vi "UIManager.Init.vi"(6 "JQMHStartup in":refnum<class "ModuleStartup.lvclass">, 8 "error in (no error)":errorcluster, 11 "NewTemplate in":refnum<class "UIManager.lvclass">) -> (0 "error out":errorcluster, 1 "StartupParams":variant, 2 "Requests":T2, 3 "NewTemplate out":refnum<class "UIManager.lvclass">, 4 "JQMHStartup out":refnum<class "ModuleStartup.lvclass">, 5 "StandardRequests":refnum<event-registration>)   [LabVIEW 2024, in "UIManager.lvclass"]
uses:
  UIManager.lvclass
  UIManager.lvclass/UIManager.ctl
  C:/Git/JA/JQMH/RQMHCore/ModuleCore/Module.lvclass
  C:/Git/JA/JQMH/ModuleTemplates/UIManager/UIManager.lvclass
  RQMHCore/Shared/ModuleShared.lvlib
  RQMHCore/ModuleCore/Module.lvclass
  RQMHCore/Startup/ModuleStartup.lvclass
  RQMHCore/ModuleCore/StopEventArgs.ctl
  Request Events--cluster.ctl
  RQMHCore/ModuleCore/StandardRequests.ctl
  RQMHCore/ModuleCore/Show Front Panel--Args.ctl
  RQMHCore/ModuleCore/Hide Front Panel.ctl
  RQMHCore/ModuleCore/Show Block Diagram.ctl
  RQMHCore/ModuleCore/Hide Block Diagram--Args.ctl
  RQMHCore/ModuleCore/Reply.ctl
  Do Something Args.ctl
  RQMHCore/ModuleCore/InitialiseArgs.ctl
  Prepare Args.ctl
  Show Args.ctl
  Add Eng Panel Args.ctl
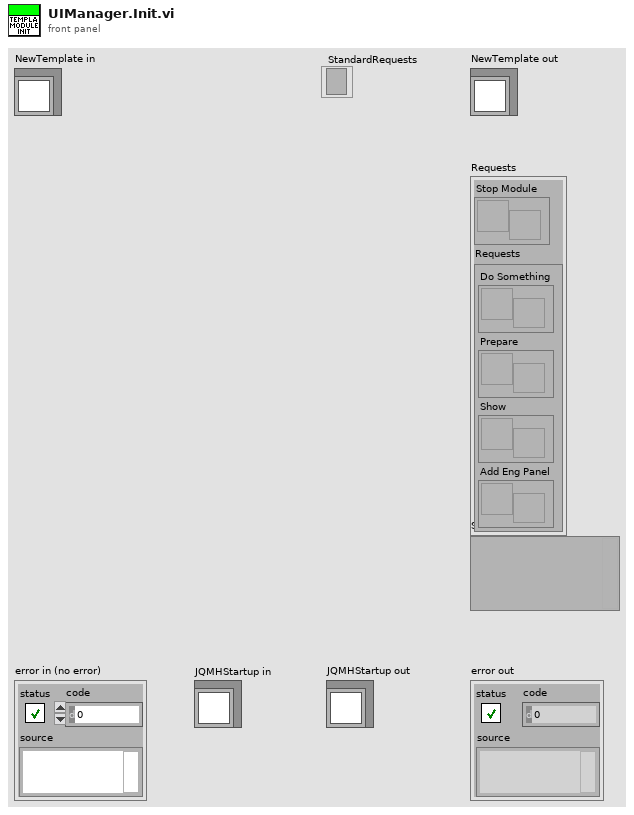
[diagram p1: front panel]
types:
  T1 = typedef "UIManager.lvclass/Request Events--cluster.ctl" = cluster{"Do Something":refnum<user-event>, "Prepare":refnum<user-event>, "Show":refnum<user-event>, "Add Eng Panel":refnum<user-event>}
  T2 = cluster{"Stop Module":refnum<user-event>, "Requests":T1}
  T3 = typedef "Module.lvclass/StandardRequests.ctl" = cluster{"Initialise":refnum<user-event>, "Stop Module":refnum<user-event>, "ShowFP":refnum<user-event>, "Hide Front Panel":refnum<user-event>, "Show Block Diagram":refnum<user-event>, "Hide Block Diagram":refnum<user-event>}
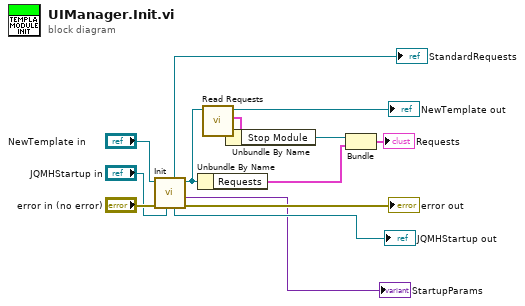
[diagram p0: block diagram]
diagram:
  n1 = call "Init.vi"("JQMHStartup.lvclass"="JQMHStartup in", "error in (no error)"="error in (no error)", "JQMHCore.lvclass"="NewTemplate in") -> ("error out"=→"error out":errorcluster, "StartupParams"=→"StartupParams":variant, "JQMHCore out"=w12:refnum<class "UIManager.lvclass">, "JQMHStartup out"=→"JQMHStartup out":refnum<class "ModuleStartup.lvclass">, "Event Registration Refnum"=→"StandardRequests":refnum<event-registration>)  [unwired: 3 in, 1 out]
  n2 = Unbundle By Name(w12) -> ("Requests"=w13:T1)
  n3 = call "Read Requests.vi"("JQMHModule in"=w12) -> ("Requests"=w5:T3, "JQMHModule out"=→"NewTemplate out":refnum<class "UIManager.lvclass">)  [unwired: 9 in]
  n4 = Unbundle By Name(w5) -> ("Stop Module"=w4:refnum<user-event>)
  n5 = Bundle("Stop Module"=w4, "Requests"=w13) -> (→"Requests":T2)  [unwired: 1 in]
